vi "Write FOAD.vi"(8 "error in (no error)":errorcluster, 10 "Father Of All Detectors.lvclass":refnum<class "Father Of All Detectors.lvclass">, 11 "Detector Manager in":refnum<class "Detector Manager.lvclass">) -> (0 "error out":errorcluster, 3 "Detector Manager out":refnum<class "Detector Manager.lvclass">)   [LabVIEW 2026, in "TALOS.lvlib" / "Detector Manager.lvlib" / "Detector Manager.lvclass"]
uses:
  Detector Manager.lvclass
  Classes/Father of all Detectors/Father Of All Detectors.lvclass
  Detector Manager.lvclass/Detector Manager.ctl
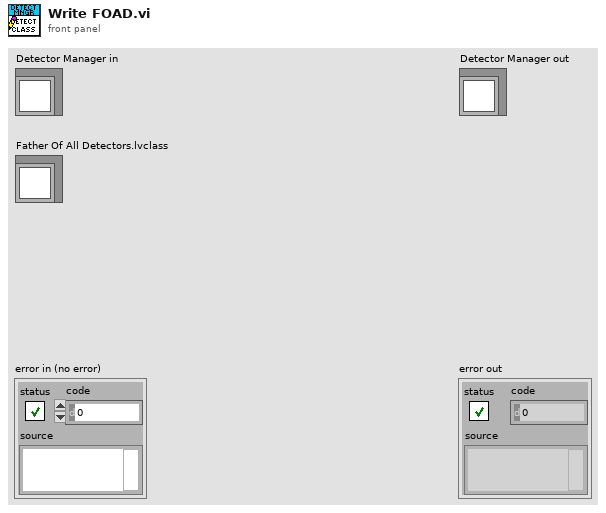
[diagram p1: front panel]
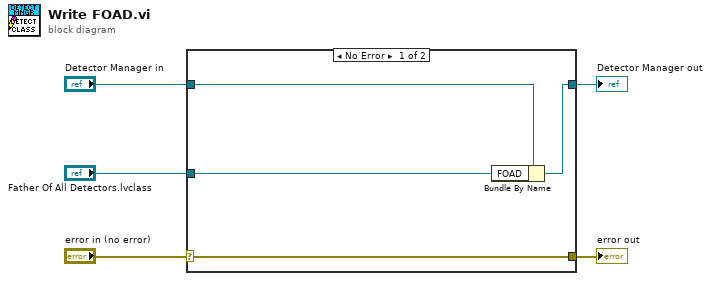
[diagram p0: block diagram]
diagram:
  n1 = case shown="No Error" "error in (no error)" {
    selector: "error in (no error)" -> [w9 w10]
    tunnel: [w9 w10] -> w4
    tunnel: [w7 w11] -> w2
    tunnel: "Detector Manager in" -> [w8 w11]
    tunnel: "Father Of All Detectors.lvclass" -> [w6 _]
    frame No Error {
      n2 = Bundle By Name(cluster=w8, "FOAD"=w6) -> (w7:refnum<class "Detector Manager.lvclass">)
    }
    frame Error {
    }
  }
  "error out" <- w4
  "Detector Manager out" <- w2
